vi "BRig_RT__Case_Exp__State_WrongOrTimeout_Pre__v2.vi"(0 "input_dataCurrent":u16[](array[numeric]), 5 "input_WorTO":bool, 7 "input_dataBlock":u16[][](array[numeric]), 9 "input_dataTrial":u16[][](array[numeric]), 11 "input_dataExp":u16[](array[numeric])) -> (1 "output_BTPR":bool, 2 "output_T2R":bool, 3 "output_T2R_or_BTPR":u16, 4 "output_dataCurrent":u16[](array[numeric]), 8 "output_dataBlock":u16[][](array[numeric]), 10 "output_dataTrial":u16[][](array[numeric]), 12 "output_avgStat":dbl, 13 "output_R(F)_or_L(T)":bool, 14 "output_sTrial_start":u16)   [LabVIEW 2014]
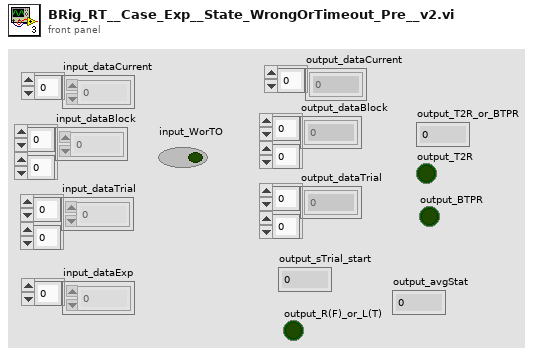
[diagram p1: front panel]
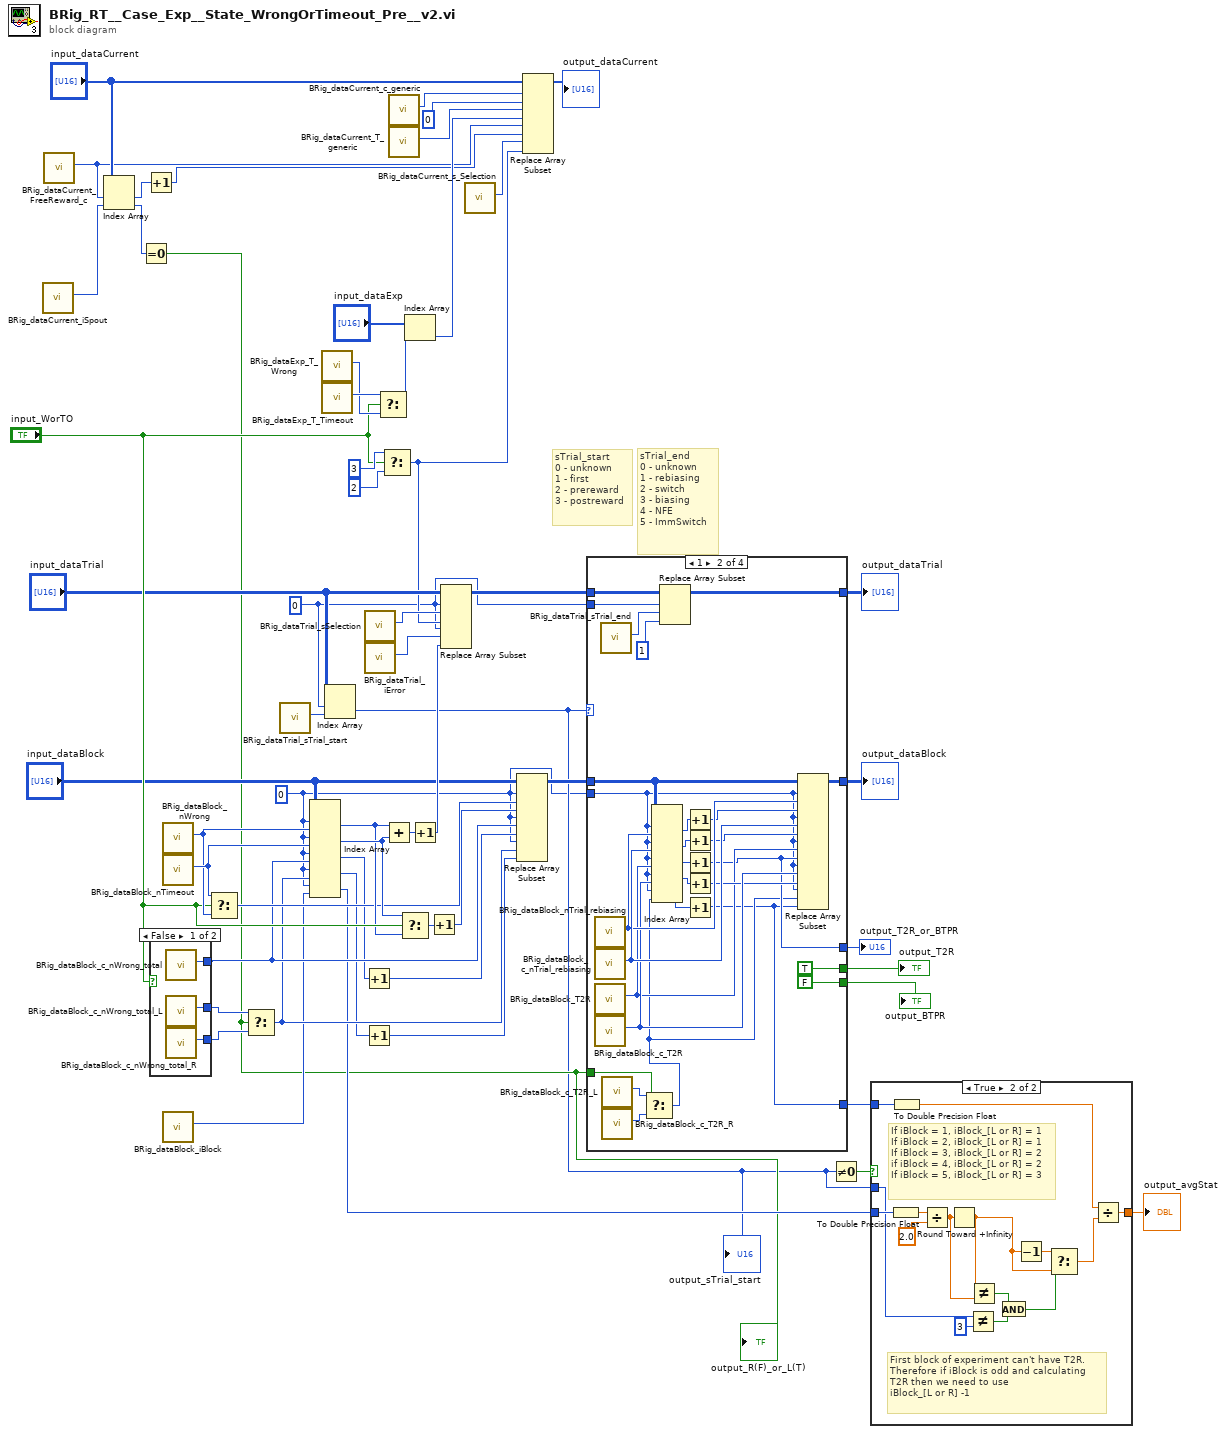
[diagram p0: block diagram]
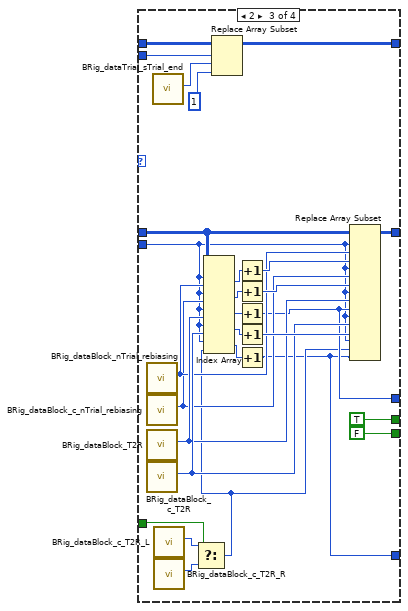
[diagram p4: hidden frame]
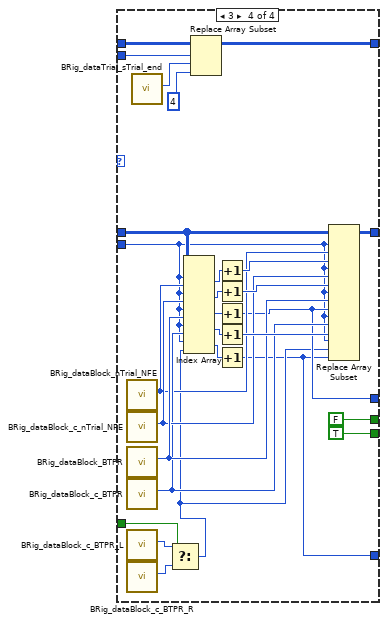
[diagram p5: hidden frame]
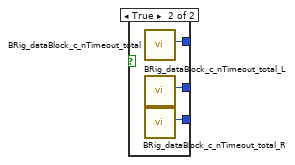
[diagram p6: hidden frame]
diagram:
  w3 = 0
  w4 = 0
  # "sTrial_end\n0 - unknown\n1 - rebiasing\n2 - switch\n3 - biasing\n4 - NFE\n5 - ImmSwitch"
  # "sTrial_start\n0 - unknown\n1 - first\n2 - prereward\n3 - postreward"
  n1 = call "BRig_dataCurrent_iSpout.vi"() -> ("output_iSpout"=w2:i32)  [unwired: 11 in]
  n2 = call "BRig_dataCurrent_FreeReward_c.vi"() -> ("output_FreeReward_c"=w18:i32)  [unwired: 11 in]
  n3 = Index Array(array="input_dataCurrent", index #1=w18, index #2=w2) -> (element #1=w19:u16, element #2=w1:u16)
  n4 = Equal To 0?(x=w1) -> (x = 0?=w7:bool)
  "output_R(F)_or_L(T)" <- w7
  n5 = Increment(x=w19) -> (x+1=w17:u16)
  n6 = case shown="False" "input_WorTO" {
    tunnel: [w61 w64] -> w31
    tunnel: [w60 w63] -> w44
    tunnel: [w59 w62] -> w43
    frame False {
      n7 = call "BRig_dataBlock_c_nWrong_total.vi"() -> ("output_c_nWrong_total"=w61:i32)  [unwired: 11 in]
      n8 = call "BRig_dataBlock_c_nWrong_total_L.vi"() -> ("output_c_nWrong_total_L"=w60:i32)  [unwired: 11 in]
      n9 = call "BRig_dataBlock_c_nWrong_total_R.vi"() -> ("output_c_nWrong_total_R"=w59:i32)  [unwired: 11 in]
    }
    frame True {
      n10 = call "BRig_dataBlock_c_nTimeout_total.vi"() -> ("output_c_nTimeout_total"=w64:i32)  [unwired: 11 in]
      n11 = call "BRig_dataBlock_c_nTimeout_total_L.vi"() -> ("output_c_nTimeout_total_L"=w63:i32)  [unwired: 11 in]
      n12 = call "BRig_dataBlock_c_nTimeout_total_R.vi"() -> ("output_c_nTimeout_total_R"=w62:i32)  [unwired: 11 in]
    }
  }
  n13 = call "BRig_dataBlock_nWrong.vi"() -> ("output_nWrong"=w39:i32)  [unwired: 11 in]
  n14 = call "BRig_dataBlock_nTimeout.vi"() -> ("output_nTimeout"=w40:i32)  [unwired: 11 in]
  n15 = call "BRig_dataBlock_iBlock.vi"() -> ("output_iBlock"=w11:i32)  [unwired: 11 in]
  n16 = Select(t=w40, s="input_WorTO", f=w39) -> (s? t:f=w33:i32)
  n17 = Select(t=w44, s=w7, f=w43) -> (s? t:f=w30:i32)
  n18 = call "BRig_dataTrial_sTrial_start.vi"() -> ("output_sTrial_start"=w25:i32)  [unwired: 11 in]
  n19 = Index Array(array="input_dataBlock", index (row) #1=w3, index (col) #1=w39, index (row) #2=w3, index (col) #2=w40, index (row) #3=w3, index (col) #3=w31, index (row) #4=w3, index (col) #4=w30, index (row) #5=w3, index (col) #5=w11) -> (element #1=w36:u16, element #2=w37:u16, element #3=w29:u16, element #4=w28:u16, element #5=w8:u16)
  n20 = call "BRig_dataExp_T_Wrong.vi"() -> ("output_T_Wrong"=w50:i32)  [unwired: 11 in]
  n21 = call "BRig_dataExp_T_Timeout.vi"() -> ("output_T_Timeout"=w51:i32)  [unwired: 11 in]
  n22 = Index Array(array="input_dataTrial", index (row)=w4, index (col)=w25) -> (element=w5:u16)
  "output_sTrial_start" <- w5
  n23 = Increment(x=w29) -> (x+1=w27:u16)
  n24 = Increment(x=w28) -> (x+1=w26:u16)
  n25 = call "BRig_dataTrial_sSelection.vi"() -> ("output_sSelection"=w46:i32)  [unwired: 11 in]
  n26 = call "BRig_dataTrial_iError.vi"() -> ("output_iError"=w45:i32)  [unwired: 11 in]
  n27 = Select(t=w51, s="input_WorTO", f=w50) -> (s? t:f=w52:i32)
  n28 = Select(t=u16 3 ("new element/subarray"), s="input_WorTO", f=u16 2 ("new element/subarray")) -> (s? t:f=w15:u16)
  n29 = Add(x=w36, y=w37) -> (x+y=w42:u16)
  n30 = call "BRig_dataCurrent_c_generic.vi"() -> ("output_count_generic"=w57:i32)  [unwired: 11 in]
  n31 = call "BRig_dataCurrent_T_generic.vi"() -> ("output_T_generic"=w56:i32)  [unwired: 11 in]
  n32 = Select(t=w37, s="input_WorTO", f=w36) -> (s? t:f=w35:u16)
  n33 = Index Array(array="input_dataExp", index=w52) -> (element=w49:u16)
  n34 = Increment(x=w42) -> (x+1=w41:u16)
  n35 = Increment(x=w35) -> (x+1=w32:u16)
  n36 = Replace Array Subset(array="input_dataTrial", new element #1=w15, index (row) #1=w4, index (col) #1=w46, new element #2=w41, index (row) #2=w4, index (col) #2=w45) -> (w23:u16[][])
  n37 = call "BRig_dataCurrent_s_Selection.vi"() -> ("output_s_Selection"=w16:i32)  [unwired: 11 in]
  n38 = Replace Array Subset(array="input_dataBlock", new element #1=w32, index (row) #1=w3, index (col) #1=w33, new element #2=w27, index (row) #2=w3, index (col) #2=w31, new element #3=w26, index (row) #3=w3, index (col) #3=w30) -> (w22:u16[][])
  n39 = Replace Array Subset(array="input_dataCurrent", new element #1=u16 0 ("new element/subarray"), index #1=w57, new element #2=w49, index #2=w56, new element #3=w17, index #3=w18, new element #4=w15, index #4=w16) -> (→"output_dataCurrent":u16[])
  n40 = case shown="1" w5 {
    tunnel: w23 -> [w66 w94 w122 w150]
    tunnel: w4 -> [_ w92 w120 w148]
    tunnel: [w66 w93 w121 w149] -> w20
    tunnel: w22 -> [w65 w83 w106 w138]
    tunnel: [w65 w82 w105 w137] -> w21
    tunnel: w3 -> [_ w69 w98 w129]
    tunnel: [_ w74 w104 w130] -> w14
    tunnel: [_ TRUE TRUE FALSE] -> w13
    tunnel: [_ FALSE FALSE TRUE] -> w12
    tunnel: w7 -> [_ w73 w96 w128]
    tunnel: [_ w67 w95 w123] -> w9
    frame 0, Default {
    }
    frame 1 {
      n41 = call "BRig_dataBlock_nTrial_rebiasing.vi"() -> ("output_nTrial_rebiasing"=w88:i32)  [unwired: 11 in]
      n42 = call "BRig_dataBlock_c_nTrial_rebiasing.vi"() -> ("output_c_nTrial_rebiasing"=w89:i32)  [unwired: 11 in]
      n43 = call "BRig_dataBlock_T2R.vi"() -> ("output_T2R"=w77:i32)  [unwired: 11 in]
      n44 = call "BRig_dataBlock_c_T2R.vi"() -> ("output_c_T2R"=w79:i32)  [unwired: 11 in]
      n45 = call "BRig_dataTrial_sTrial_end.vi"() -> ("output_sTrial_end"=w91:i32)  [unwired: 11 in]
      n46 = call "BRig_dataBlock_c_T2R_L.vi"() -> ("output_c_T2R_L"=w72:i32)  [unwired: 11 in]
      n47 = call "BRig_dataBlock_c_T2R_R.vi"() -> ("output_c_T2R_R"=w71:i32)  [unwired: 11 in]
      n48 = Select(t=w72, s=w73, f=w71) -> (s? t:f=w68:i32)
      n49 = Index Array(array=w83, index (row) #1=w69, index (col) #1=w88, index (row) #2=w69, index (col) #2=w89, index (row) #3=w69, index (col) #3=w77, index (row) #4=w69, index (col) #4=w79, index (row) #5=w69, index (col) #5=w68) -> (element #1=w87:u16, element #2=w85:u16, element #3=w81:u16, element #4=w80:u16, element #5=w70:u16)
      n50 = Replace Array Subset(array=w94, new element=u16 1 ("new element/subarray"), index (row)=w92, index (col)=w91) -> (w93:u16[][])
      n51 = Increment(x=w87) -> (x+1=w86:u16)
      n52 = Increment(x=w85) -> (x+1=w84:u16)
      n53 = Increment(x=w81) -> (x+1=w74:u16)
      n54 = Increment(x=w80) -> (x+1=w78:u16)
      n55 = Increment(x=w70) -> (x+1=w67:u16)
      n56 = Replace Array Subset(array=w83, new element #1=w86, index (row) #1=w69, index (col) #1=w88, new element #2=w84, index (row) #2=w69, index (col) #2=w89, new element #3=w74, index (row) #3=w69, index (col) #3=w77, new element #4=w78, index (row) #4=w69, index (col) #4=w79, new element #5=w67, index (row) #5=w69, index (col) #5=w68) -> (w82:u16[][])
    }
    frame 2 {
      n57 = call "BRig_dataBlock_nTrial_rebiasing.vi"() -> ("output_nTrial_rebiasing"=w108:i32)  [unwired: 11 in]
      n58 = call "BRig_dataBlock_c_nTrial_rebiasing.vi"() -> ("output_c_nTrial_rebiasing"=w107:i32)  [unwired: 11 in]
      n59 = call "BRig_dataBlock_T2R.vi"() -> ("output_T2R"=w115:i32)  [unwired: 11 in]
      n60 = call "BRig_dataBlock_c_T2R.vi"() -> ("output_c_T2R"=w116:i32)  [unwired: 11 in]
      n61 = call "BRig_dataTrial_sTrial_end.vi"() -> ("output_sTrial_end"=w119:i32)  [unwired: 11 in]
      n62 = call "BRig_dataBlock_c_T2R_L.vi"() -> ("output_c_T2R_L"=w101:i32)  [unwired: 11 in]
      n63 = call "BRig_dataBlock_c_T2R_R.vi"() -> ("output_c_T2R_R"=w100:i32)  [unwired: 11 in]
      n64 = Select(t=w101, s=w96, f=w100) -> (s? t:f=w97:i32)
      n65 = Index Array(array=w106, index (row) #1=w98, index (col) #1=w108, index (row) #2=w98, index (col) #2=w107, index (row) #3=w98, index (col) #3=w115, index (row) #4=w98, index (col) #4=w116, index (row) #5=w98, index (col) #5=w97) -> (element #1=w109:u16, element #2=w111:u16, element #3=w113:u16, element #4=w114:u16, element #5=w99:u16)
      n66 = Replace Array Subset(array=w122, new element=u16 1 ("new element/subarray"), index (row)=w120, index (col)=w119) -> (w121:u16[][])
      n67 = Increment(x=w109) -> (x+1=w110:u16)
      n68 = Increment(x=w111) -> (x+1=w112:u16)
      n69 = Increment(x=w113) -> (x+1=w104:u16)
      n70 = Increment(x=w114) -> (x+1=w117:u16)
      n71 = Increment(x=w99) -> (x+1=w95:u16)
      n72 = Replace Array Subset(array=w106, new element #1=w110, index (row) #1=w98, index (col) #1=w108, new element #2=w112, index (row) #2=w98, index (col) #2=w107, new element #3=w104, index (row) #3=w98, index (col) #3=w115, new element #4=w117, index (row) #4=w98, index (col) #4=w116, new element #5=w95, index (row) #5=w98, index (col) #5=w97) -> (w105:u16[][])
    }
    frame 3 {
      n73 = call "BRig_dataBlock_nTrial_NFE.vi"() -> ("output_nTrial_NFE"=w133:i32)  [unwired: 11 in]
      n74 = call "BRig_dataBlock_c_nTrial_NFE.vi"() -> ("output_c_nTrial_NFE"=w135:i32)  [unwired: 11 in]
      n75 = call "BRig_dataBlock_BTPR.vi"() -> ("output_BTPR"=w136:i32)  [unwired: 11 in]
      n76 = call "BRig_dataBlock_c_BTPR.vi"() -> ("output_c_BTPR"=w134:i32)  [unwired: 11 in]
      n77 = call "BRig_dataBlock_c_BTPR_L.vi"() -> ("output_c_BTPR_L"=w127:i32)  [unwired: 11 in]
      n78 = call "BRig_dataBlock_c_BTPR_R.vi"() -> ("output_c_BTPR_R"=w126:i32)  [unwired: 11 in]
      n79 = call "BRig_dataTrial_sTrial_end.vi"() -> ("output_sTrial_end"=w147:i32)  [unwired: 11 in]
      n80 = Select(t=w127, s=w128, f=w126) -> (s? t:f=w124:i32)
      n81 = Index Array(array=w138, index (row) #1=w129, index (col) #1=w133, index (row) #2=w129, index (col) #2=w135, index (row) #3=w129, index (col) #3=w136, index (row) #4=w129, index (col) #4=w134, index (row) #5=w129, index (col) #5=w124) -> (element #1=w139:u16, element #2=w141:u16, element #3=w143:u16, element #4=w144:u16, element #5=w125:u16)
      n82 = Replace Array Subset(array=w150, new element=u16 4 ("new element/subarray"), index (row)=w148, index (col)=w147) -> (w149:u16[][])
      n83 = Increment(x=w139) -> (x+1=w140:u16)
      n84 = Increment(x=w141) -> (x+1=w142:u16)
      n85 = Increment(x=w143) -> (x+1=w130:u16)
      n86 = Increment(x=w144) -> (x+1=w145:u16)
      n87 = Increment(x=w125) -> (x+1=w123:u16)
      n88 = Replace Array Subset(array=w138, new element #1=w140, index (row) #1=w129, index (col) #1=w133, new element #2=w142, index (row) #2=w129, index (col) #2=w135, new element #3=w130, index (row) #3=w129, index (col) #3=w136, new element #4=w145, index (row) #4=w129, index (col) #4=w134, new element #5=w123, index (row) #5=w129, index (col) #5=w124) -> (w137:u16[][])
    }
  }
  "output_dataBlock" <- w21
  "output_dataTrial" <- w20
  "output_T2R_or_BTPR" <- w14
  "output_T2R" <- w13
  "output_BTPR" <- w12
  n89 = Not Equal To 0?(x=w5) -> (x != 0?=w10:bool)
  n90 = case shown="True" w10 {
    tunnel: w9 -> [_ w165]
    tunnel: w8 -> [_ w164]
    tunnel: [_ w160] -> w6
    tunnel: w5 -> [_ w158]
    frame False {
    }
    frame True {
      # "First block of experiment can't have T2R.\nTherefore if iBlock is odd and calculating\nT2R then we need to use\niBlock_[L or R] -1"
      # "If iBlock = 1, iBlock_[L or R] = 1\nIf iBlock = 2, iBlock_[L or R] = 1\nIf iBlock = 3, iBlock_[L or R] = 2\nif iBlock = 4, iBlock_[L or R] = 2\nIf iBlock = 5, iBlock_[L or R] = 3"
      n91 = To Double Precision Float(number=w164) -> (double precision float=w163:dbl)
      n92 = To Double Precision Float(number=w165) -> (double precision float=w161:dbl)
      n93 = Divide(x=w163, y=2.0) -> (x/y=w159:dbl)
      n94 = Round Toward +Infinity(x=w159) -> (ceil(x): smallest int >= x=w152:dbl)
      n95 = Not Equal?(x=w158, y=u16 3) -> (x != y?=w155:bool)
      n96 = Not Equal?(x=w152, y=w159) -> (x != y?=w156:bool)
      n97 = And(x=w156, y=w155) -> (x .and. y?=w154:bool)
      n98 = Decrement(x=w152) -> (x-1=w153:dbl)
      n99 = Select(t=w153, s=w154, f=w152) -> (s? t:f=w151:dbl)
      n100 = Divide(x=w161, y=w151) -> (x/y=w160:dbl)
    }
  }
  "output_avgStat" <- w6
